vi "Time delay - OFF (SubVI).vi"(7 "Toff":dbl) -> (1 "Output":dbl)   [LabVIEW 2016]
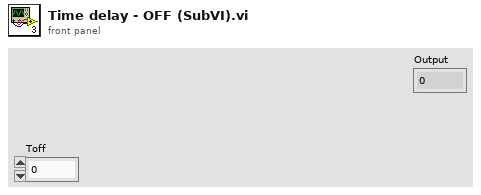
[diagram p1: front panel]
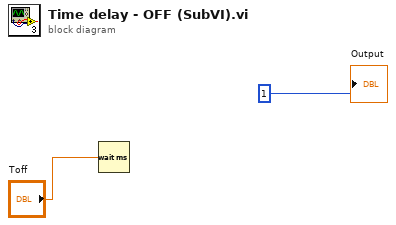
[diagram p0: block diagram]
diagram:
  n1 = Wait (ms)(milliseconds to wait="Toff") -> ()  [unwired: 1 out]
  "Output" <- 1
